vi "Daemon.vi"() -> ()   [LabVIEW 2013]
uses:
  <vilib>/NI/AMC/Read Termination Message.vi
  <vilib>/NI/AMC/Create Single Message.vi
  <vilib>/NI/AMC/Update Message Routing Info.vi
  <vilib>/NI/AMC/Send Message.vi
  <vilib>/NI/AMC/Globals.vi
  <vilib>/NI/AMC/AMC.lvlib
panel:
  out "source process":string
  out "Message Value":dbl
  out "status":string
  in  "process":bool
  in  "exit":bool
  in  "state variables":cluster{"CurrentFile":path}
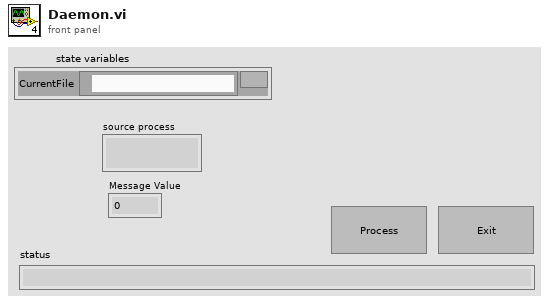
[diagram p1: front panel]
types:
  T1 = typedef "AMC.lvlib/Message Queue.ctl" = refnum<queue>
  T2 = typedef "AMC.lvlib/Message.ctl" = cluster{"name":string, "value":string, "attributes":T3, "receiver host":string, "receiver process":string, "source host":string, "source process":string, "priority message":bool, "acknowledge message":bool}
  T3 = typedef "Tools_KeyedArray.lvlib/KeyedArray.ctl" = cluster{"keys":string[], "values":string[]}
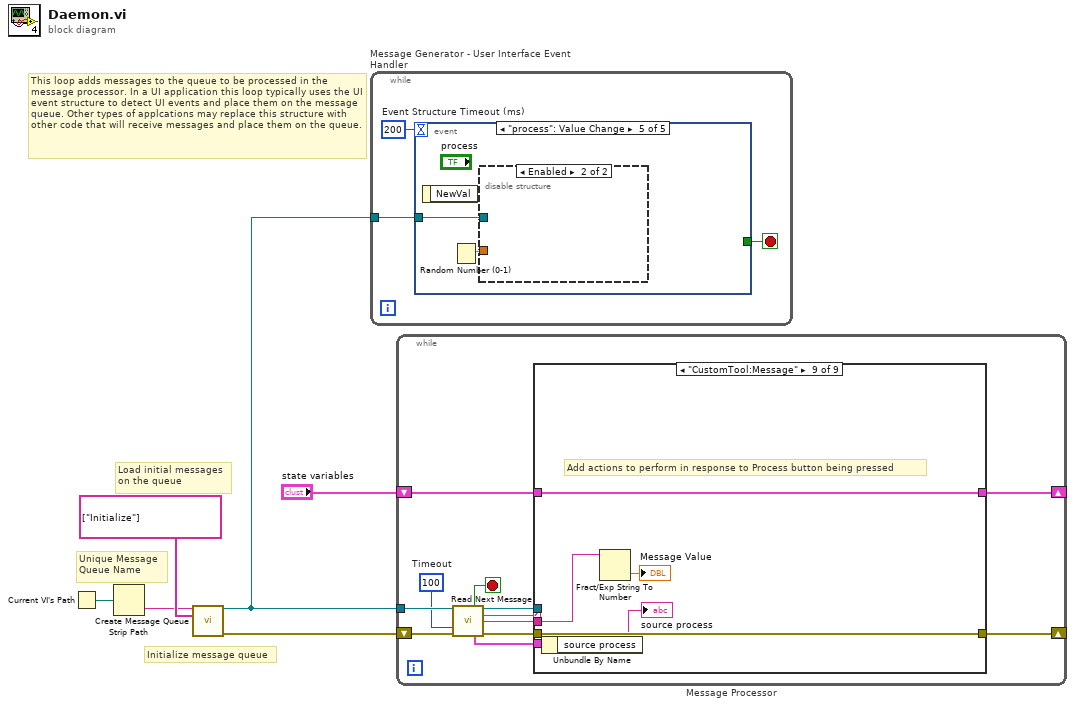
[diagram p0: block diagram]
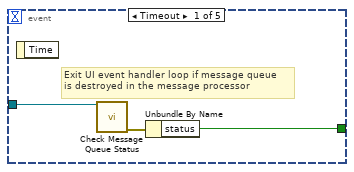
[diagram p2: hidden frame]
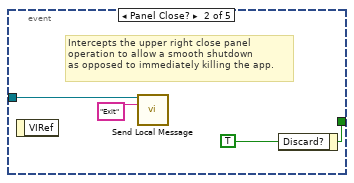
[diagram p3: hidden frame]
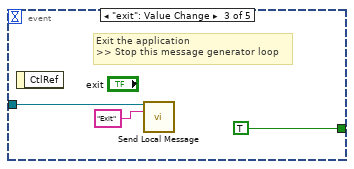
[diagram p4: hidden frame]
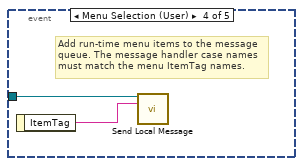
[diagram p5: hidden frame]
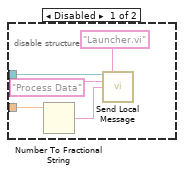
[diagram p6: hidden frame]
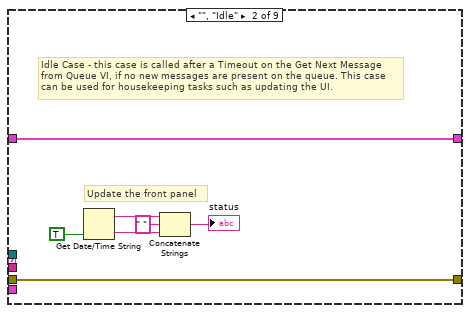
[diagram p8: hidden frame]
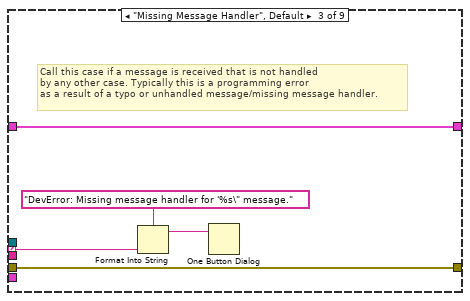
[diagram p9: hidden frame]
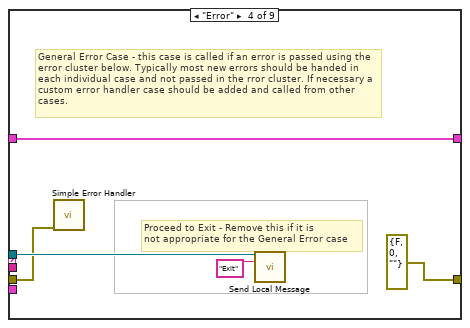
[diagram p10: hidden frame]
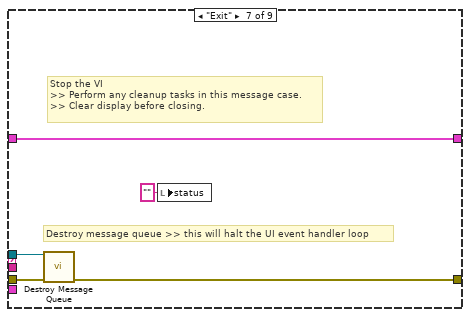
[diagram p13: hidden frame]
diagram:
  # "This loop adds messages to the queue to be processed in the message processor. In a UI application this loop typically uses the UI event structure to detect UI events and place them on the message queue. Other types of applcations may replace this structure with other code that will receive messages and place them on the queue."
  # "Initialize message queue"
  # "Unique Message\nQueue Name"
  # "Load initial messages\non the queue"
  n1 = Current VI's Path() -> (path=w1:path)
  n2 = Strip Path(path=w1) -> (name=w5:string)  [unwired: 1 out]
  n3 = call <vilib>:"Create Message Queue.vi"("message queue name"=w5, "initial message names"=string[] ["Initialize"]) -> ("message queue out"=w4:T1, "error out"=w3:errorcluster)  [unwired: 12 in]
  n4 = while "Message Generator - User Interface Event Handler" {
    tunnel: w4 -> [w7]
    stop <- w8 stop-if-true
    w9 = 200  # Event Structure Timeout (ms)
    n5 = event shown="[4] \"process\": Value Change" {
      selector: _ -> [_ _ _ _ _]
      dyn-events: _ -> [_ _ _ _ _]
      timeout: w9 -> [_ _ _ _ _]
      tunnel: [w10 w15 TRUE ("Discard?") _ _] -> w8
      tunnel: w7 -> [w11 w13 w16 w19 w22]
      event Timeout {
        # "Exit UI event handler loop if message queue\nis destroyed in the message processor"
        n6 = event-data() -> ()  [unwired: 2 out]
        n7 = call <vilib>:"Check Message Queue Status.vi"("message queue in"=w11) -> ("error out"=w12:errorcluster)  [unwired: 10 in, 4 out]
        n8 = Unbundle By Name(w12) -> ("status"=w10:bool)
      }
      event Panel Close? {
        w15 = TRUE ("Discard?")
        # "Intercepts the upper right close panel\noperation to allow a smooth shutdown\nas opposed to immediately killing the app."
        n9 = event-data() -> ()  [unwired: 2 out]
        n10 = call <vilib>:"Send Local Message.vi"("message queue in"=w13, "message name"="Exit") -> ()  [unwired: 11 in, 3 out]
        n11 = event-data("Discard?"=w15) -> ()  [unwired: 1 in, 1 out]
      }
      event "exit": Value Change {
        # "Exit the application\n>> Stop this message generator loop"
        n12 = event-data() -> ()  [unwired: 2 out]
        n13 = call <vilib>:"Send Local Message.vi"("message queue in"=w16, "message name"="Exit") -> ()  [unwired: 11 in, 3 out]
      }
      event Menu Selection (User) {
        # "Add run-time menu items to the message\nqueue. The message handler case names must match the menu ItemTag names."
        n14 = event-data() -> ("ItemTag"=w20:string)  [unwired: 1 out]
        n15 = call <vilib>:"Send Local Message.vi"("message queue in"=w19, "message name"=w20) -> ()  [unwired: 11 in, 3 out]
      }
      event "process": Value Change {
        n16 = event-data() -> ()  [unwired: 2 out]
        n17 = Random Number (0-1)() -> (number: 0 to 1=w21:dbl)
        n18 = disable-structure shown="Enabled" {
          disable-tunnel: w22 -> [w27 _]
          disable-tunnel: w21 -> [w24 _]
          frame Disabled {
            n19 = Number To Fractional String(number=w24) -> (F-format string=w25:string)  [unwired: 3 out]
            n20 = call <vilib>:"Send Local Message.vi"("message queue in"=w27, "receiver process (\"\" - local)"="Launcher.vi" ("receiver process (\"\" - local)"), "message name"="Process Data", "message value"=w25) -> ()  [unwired: 9 in, 3 out]
          }
          frame Enabled {
          }
        }
      }
    }
  }
  n21 = while "Message Processor" {
    shift-left: w3 -> [w33]
    shift-right: [w37] -> _
    tunnel: w4 -> [w34]
    shift-left: "state variables" -> [w39]
    shift-right: [w38] -> _
    stop <- w36 stop-if-true
    w29 = 100  # Timeout
    n22 = call <vilib>:"Read Next Message.vi"("message queue in"=w34, "timeout (1 ms)"=w29, "error in"=w33) -> ("exit process?"=w36:bool, "message queue out"=w35:T1, "message name"=w31:string, "message value"=w30:string, "message"=w28:T2, "error out"=w32:errorcluster)  [unwired: 5 in, 2 out]
    n23 = case shown="\"CustomTool:Message\"" w31 {
      selector: w31 -> [_ _ w51 _ _ _ _ _ _]
      tunnel: [w41 w48 w53 w58 w60 w62 w67 w69 w74] -> w38
      tunnel: w39 -> [w41 w48 w53 w58 w60 w62 w67 w69 w74]
      tunnel: w35 -> [_ _ _ w56 _ _ w64 _ _]
      tunnel: w32 -> [w40 w47 w52 w54 w59 w61 w65 w68 w75]
      tunnel: [w40 w47 w52 errorcluster {"status"=FALSE, "code"=0, "source"=""} ("error out") w59 w61 w63 w68 w75] -> w37
      tunnel: w30 -> [_ _ _ _ _ _ _ _ w73]
      tunnel: w28 -> [_ _ _ _ _ _ _ _ w71]
      frame "---------- Framework Operations ----------" {
        # "Dummy case to add a seperator in the Case Structure menu"
      }
      frame "", "Idle" {
        # "Update the front panel"
        # "Idle Case - this case is called after a Timeout on the Get Next Message from Queue VI, if no new messages are present on the queue. This case can be used for housekeeping tasks such as updating the UI."
        n24 = Get Date/Time String(want seconds? (F)=TRUE) -> (date string=w46:string, time string=w45:string)  [unwired: 2 out]
        n25 = Concatenate Strings(w46, " " ("string"), w45) -> (→"status":string)
      }
      frame "Missing Message Handler", Default {
        # "Call this case if a message is received that is not handled \nby any other case. Typically this is a programming error\nas a result of a typo or unhandled message/missing message handler."
        n26 = Format Into String(format string="DevError: Missing message handler for '%s\" message." ("message"), w51) -> (resulting string=w49:string)  [unwired: 2 in, 1 out]
        n27 = One Button Dialog(message=w49) -> ()  [unwired: 2 out]
      }
      frame "Error" {
        # "Proceed to Exit - Remove this if it is\nnot appropriate for the General Error case"
        # "General Error Case - this case is called if an error is passed using the error cluster below. Typically most new errors should be handed in each individual case and not passed in the rror cluster. If necessary a custom error handler case should be added and called from other cases."
        n28 = call <vilib>:"Simple Error Handler.vi"("error in (no error)"=w54) -> ()  [unwired: 1 in, 8 out]
        n29 = call <vilib>:"Send Local Message.vi"("message queue in"=w56, "message name"="Exit") -> ()  [unwired: 11 in, 3 out]
      }
      frame "---------- Generic Operations ----------" {
        # "Dummy case to add a seperator in the Case Structure menu"
      }
      frame "Initialize" {
        # "Initialize the state variables and user interface"
      }
      frame "Exit" {
        # "Destroy message queue >> this will halt the UI event handler loop"
        # "Stop the VI\n>> Perform any cleanup tasks in this message case.\n>> Clear display before closing."
        n30 = call <vilib>:"Destroy Message Queue.vi"("message queue in"=w64, "error in"=w65) -> ("error out"=w63:errorcluster)  [unwired: 11 in, 2 out]
        n31 = local write "status"("" ("Status")) -> ()
      }
      frame "---------- Application Operations ----------" {
        # "Dummy case to add a seperator in the Case Structure menu"
      }
      frame "CustomTool:Message" {
        # "Add actions to perform in response to Process button being pressed"
        n32 = Unbundle By Name(w71) -> ("source process"=→"source process":string)
        n33 = Fract/Exp String To Number(string=w73) -> (number=→"Message Value":dbl)  [unwired: 4 out]
      }
    }
  }
